vi "Get DDS Cur Boxing Bias Mv Min.vi"(8 "error in (no error)":errorcluster, 11 "boxing":u32) -> (0 "error out":errorcluster, 3 "function return":i32)   [LabVIEW 2023, in "vmmsolib.lvlib"]
doc: "DLL_API int WINAPI GetDDSCurBoxingBiasMvMin(unsigned int boxing);"
uses:
  vmmsolib.lvlib
  vmmso.dll
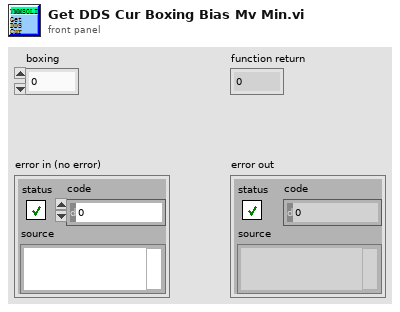
[diagram p1: front panel]
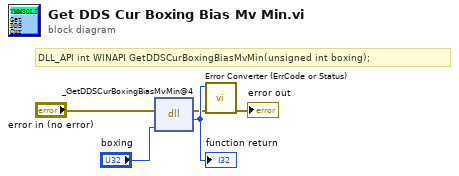
[diagram p0: block diagram]
diagram:
  # "DLL_API int WINAPI GetDDSCurBoxingBiasMvMin(unsigned int boxing);"
  n1 = dll-call lib="D:/VmMsoSDK/demo-Labview/2023/vmmsolib/vmmso.*" fn="_GetDDSCurBoxingBiasMvMin@4"(error in="error in (no error)", "boxing"="boxing") -> (error out=w2:errorcluster, w5:i32)  [unwired: 3 in, 1 out]
  "function return" <- w5
  n2 = call "Error Converter (ErrCode or Status).vi"("error in (no error)"=w2, "error code"=w5) -> ("error out"=→"error out":errorcluster)  [unwired: 9 in]
